vi "Comm Connection Engine.vi"(8 "error in (no error)":errorcluster, 10 "Comm.lvclass":refnum<class "VeriStand Comm.lvclass">, 11 "Process":refnum<class "Process.lvclass">) -> (0 "error out":errorcluster)   [LabVIEW 2015, in "NI VeriStand Addon Network Comm.lvlib" / "VeriStand Comm.lvclass"]
uses:
  VeriStand Comm.lvclass
  <vilib>/NI/NI VeriStand Inline Async API/_VS Inline Async API/Process/Process.lvclass
  VeriStand Comm.lvclass/VeriStand Comm.ctl
  <vilib>/NI/STM/TCP/TCP Read Options.ctl
  <vilib>/NI/STM/Connection Manager/TCP/TCP Connection Method.ctl
  <vilib>/NI/STM/Connection Manager/TCP/TCP Connection Properties.ctl
  <vilib>/NI/NI VeriStand Inline Async API/_VS Inline Async API/Process/Process.lvclass/Process.ctl
  <vilib>/NI/STM/TCP/Get Connection Reference (TCP).vi
  <vilib>/NI/STM/TCP/Read Meta Data (TCP Ref).vi
  <vilib>/NI/NI VeriStand Inline Async API/_VS Inline Async API/Error Handling Process/SubVIs/Error.ConvertArray.vi
  <vilib>/NI/STM/TCP/Read Meta Data (TCP Clst).vi
  <vilib>/NI Veristand/Custom Device Tools/Custom Device Utility Library/Custom Device Utility Library.lvlib
  <vilib>/NI/STM/NI STM.lvlib
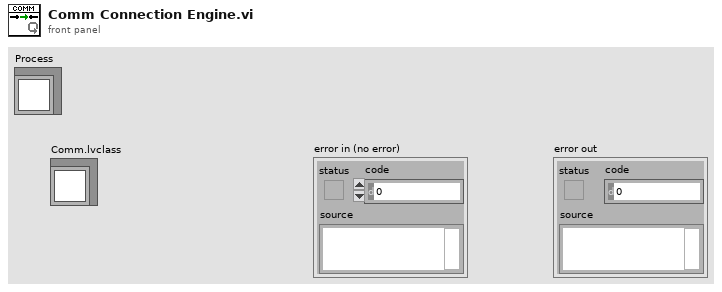
[diagram p1: front panel]
types:
  T1 = typedef "TCP Connection Manager Reference.ctl" = refnum<data-value>
  T2 = typedef "NI STM.lvlib/TCP Read Options.ctl" = cluster{"ignore timeout error":bool, "timeout ms (1000)":i32}
  T3 = typedef "NI STM.lvlib/TCP Connection Properties.ctl" = cluster{"Name":string, "Address":string, "Custom":string}
  T4 = typedef "NI STM.lvlib/TCP Connection Method.ctl" = enum16{"Initialize", "Add Connection", "Set Properties", "Get Connection(s)", "Remove Connection", "Remove All Connections", "Get Connection Count"}
  T5 = typedef "NI STM.lvlib/TCP Connection Info.ctl" = cluster{"connection ID":refnum<k5>, "meta data":T6[]}
  T6 = typedef "NI STM.lvlib/MetaDataElement.ctl" = string
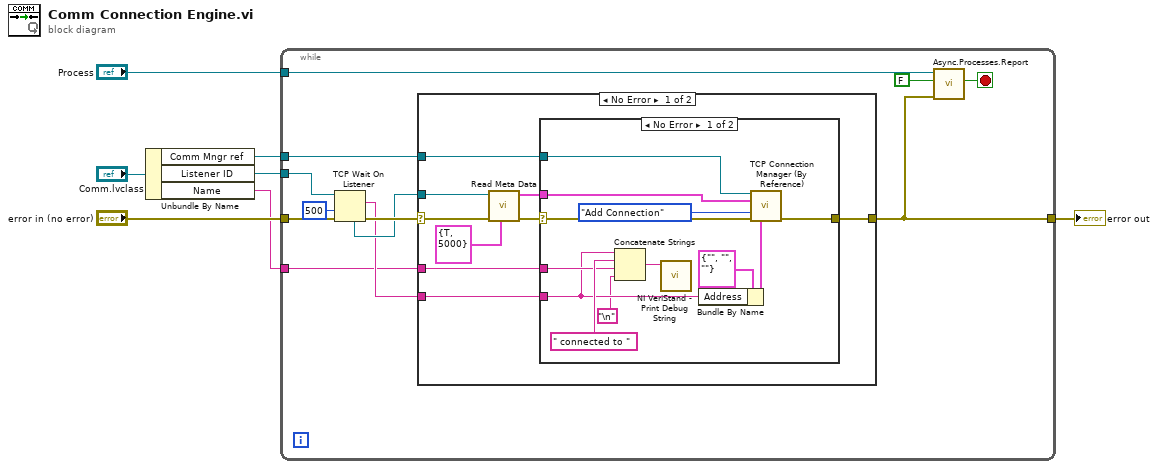
[diagram p0: block diagram]
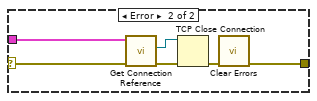
[diagram p2: hidden frame]
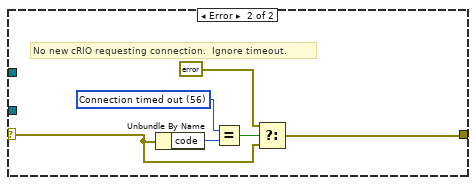
[diagram p3: hidden frame]
diagram:
  n1 = Unbundle By Name("Comm.lvclass") -> ("Comm Mngr ref"=w6:T1, "Listener ID"=w7:refnum<k5>, "Name"=w2:string)
  n2 = while {
    tunnel: "error in (no error)" -> [w19]
    tunnel: w7 -> [w18]
    tunnel: "Process" -> [w12]
    tunnel: [w8] -> w3
    tunnel: w6 -> [w10]
    tunnel: w2 -> [w9]
    stop <- w13 stop-if-true
    n3 = TCP Wait On Listener(8:w19, 9:500 ("timeout ms (wait forever: -1)"), 11:w18) -> (0:w16:errorcluster, 2:w14:string, 4:w15:refnum<k5>)  [unwired: 1 in, 2 out]
    n4 = case shown="No Error" w16 {
      selector: w16 -> [w28 w48]
      tunnel: w15 -> [w23 _]
      tunnel: [w27 w49] -> w8
      tunnel: w14 -> [w25 _]
      tunnel: w10 -> [w26 _]
      tunnel: w9 -> [w24 _]
      frame No Error {
        n5 = call-poly <vilib>:"Read Meta Data.vi"("options"=T2 {"ignore timeout error"=TRUE, "timeout ms (1000)"=5000}, "error in"=w28, "connection ID"=w23) -> ("error out"=w22:errorcluster, "connection info out"=w21:T5)  [unwired: 6 in, 1 out]
        n6 = case shown="No Error" w22 {
          selector: w22 -> [w39 w43]
          tunnel: w26 -> [w37 _]
          tunnel: w21 -> [w38 w44]
          tunnel: [w40 w46] -> w27
          tunnel: w25 -> [w33 _]
          tunnel: w24 -> [w34 _]
          frame No Error {
            n7 = Concatenate Strings(w33, " connected to " ("string"), w34, "\n") -> (w35:string)
            n8 = call <vilib>:"NI VeriStand - Print Debug String.vi"("Message"=w35) -> ()  [unwired: 10 in, 1 out]
            n9 = Bundle By Name(cluster=T3 {"Name"="", "Address"="", "Custom"=""} ("properties in"), "Address"=w33) -> (w29:T3)
            n10 = call <vilib>:"TCP Connection Manager (By Reference).vi"("connection manager ref in"=w37, "connection in"=w38, "method"=TCP_Connection_Method."Add Connection", "error in"=w39, "properties in"=w29) -> ("error out"=w40:errorcluster)  [unwired: 4 in, 6 out]
          }
          frame Error {
            n11 = call-poly <vilib>:"Get Connection Reference.vi"("error in"=w43, "connection info in"=w44) -> ("error out"=w41:errorcluster, "connection ID out"=w42:refnum<k5>)  [unwired: 7 in, 1 out]
            n12 = TCP Close Connection(connection ID=w42, error in (no error)=w41) -> (error out=w45:errorcluster)  [unwired: 1 in, 1 out]
            n13 = call <vilib>:"Clear Errors.vi"("error in (no error)"=w45) -> ("error out"=w46:errorcluster)  [unwired: 5 in, 1 out]
          }
        }
      }
      frame Error {
        w47 = 56 items=["No Error", "Argument Error", "Memory Full", "Out of Zone", "End of File", "File Already Open", "Generic File IO Error", "File Not Found", "File Permission Error", "Disk Full", "Duplicate Path", "Too Many Files Open", "Not Enabled", "Resource File Not Found", "Cannot Add Resource", "Resource Not Found", "Image Not Found", "Image Memory Error", "Pen Does Not Exist", "Config Bad Type", "Config Token Not Found", "Config Parse Error", "Config Memory Error", "Bad External Code Format", "Bad External Code Offset", "External Code Not Present", "Null Window", "Destroy Window Mixup", "Null Menu", "Print Aborted", "Bad Print Record", "Print Driver Error", "Windows Error During Print", "Memory Error During Print", "Print Dialog Error", "Generic Print Error", "Invalid Device Refnum", "Device Not Found", "Device Parameter Error", "Device Unit Error", "Can't Open Device", "Device Call Aborted", "Generic Error", "Cancelled By User", "Object ID Too Low", "Object ID Too High", "Object Not In Heap", "Unknown Heap", "Bad DefProc ID", "DefProc Not In Table", "Message Out Of Range", "Null Method", "Unknown Message", "Manager Call Not Supported", "Bad address", "Connection In progress", "Connection timed out", "Connection is already in progress", "Network attribute not supported", "Network error", "Address in use", "System out of memory", "Connection aborted", "Connection refused", "Connection is not connected", "Connection is already connected", "Connection closed", "Initialize error (interapplication manager)", "Bad occurrence", "Wait on unbound occurrence handler", "Occurrence queue overflow", "Bad path", "Semaphore not signaled", "Unrecognized type (interapplication manager)"] ("1st Error to Convert")
        # "No new cRIO requesting connection.  Ignore timeout."
        n14 = Unbundle By Name(w48) -> ("code"=w51:i32)
        n15 = Equal?(x=w47, y=w51) -> (x = y?=w52:bool)
        n16 = Select(t=errorcluster {"status"=FALSE, "code"=0, "source"=""} ("error in (no error)"), s=w52, f=w48) -> (s? t:f=w49:errorcluster)
      }
    }
    n17 = call <vilib>:"Async.Processes.Report.vi"("Error"=w8, "Stop on Error?"=FALSE, "Process in"=w12) -> ("Stop"=w13:bool)  [unwired: 7 in, 1 out]
  }
  "error out" <- w3
